vi "Init Panels.vi"(8 "error in (no error)":errorcluster, 11 "SB App in":refnum<class "SB App.lvclass">) -> (0 "error out":errorcluster, 3 "SB App out":refnum<class "SB App.lvclass">)   [LabVIEW 2020, in "SB App.lvlib" / "SB App.lvclass"]
uses:
  SB App.lvclass
  Game Config Panel/Game Config Panel.lvclass
  C:/Program Files (x86)/National Instruments/LabVIEW 2020/vi.lib/IlluminatedG/IG OOPanel/OOPanel/Panel/Panel.lvclass
  Dashboard Panel/Dashboard Panel.lvclass
  Team Field Panel/Team Field Panel.lvclass
  Square Field Panel/Square Field Panel.lvclass
  SB App.lvclass/SB App.ctl
  <vilib>/IlluminatedG/IG OOPanel/OOPanel/Manager/Manager.lvclass
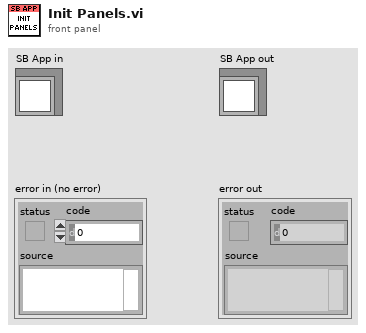
[diagram p1: front panel]
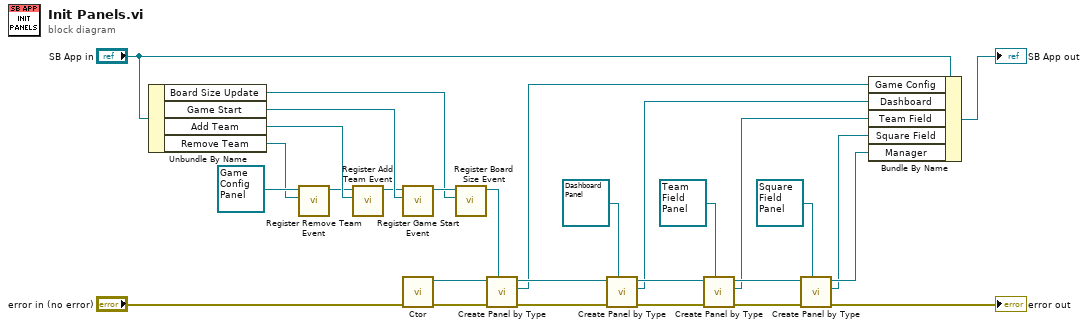
[diagram p0: block diagram]
diagram:
  n1 = Unbundle By Name("SB App in") -> ("Board Size Update"=w7:refnum<user-event>, "Game Start"=w9:refnum<user-event>, "Add Team"=w4:refnum<user-event>, "Remove Team"=w1:refnum<user-event>)
  n2 = call "Register Remove Team Event.vi"("Remove Team"=w1, "Game Config Panel in"=refnum<class "Game Config Panel.lvclass"> refnum ("SB App.lvlib:Game Config Panel.lvclass")) -> ("Game Config Panel out"=w3:refnum<class "Game Config Panel.lvclass">)  [unwired: 8 in, 1 out]
  n3 = call "Register Add Team Event.vi"("Add Team"=w4, "Game Config Panel in"=w3) -> ("Game Config Panel out"=w5:refnum<class "Game Config Panel.lvclass">)  [unwired: 8 in, 1 out]
  n4 = call "Register Game Start Event.vi"("Game Start"=w9, "Game Config Panel in"=w5) -> ("Game Config Panel out"=w8:refnum<class "Game Config Panel.lvclass">)  [unwired: 8 in, 1 out]
  n5 = call <vilib>:"Ctor.vi"("error in (no error)"="error in (no error)") -> ("error out"=w15:errorcluster, "Manager out"=w29:refnum<class "Manager.lvclass">)  [unwired: 9 in]
  n6 = call "Register Board Size Event.vi"("Board Size Update"=w7, "Game Config Panel in"=w8) -> ("Game Config Panel out"=w6:refnum<class "Game Config Panel.lvclass">)  [unwired: 8 in, 1 out]
  n7 = call <vilib>:"Create Panel by Type.vi"("Panel Type"=w6, "error in (no error)"=w15, "Manager in"=w29) -> ("error out"=w14:errorcluster, "Panel"=w18:refnum<class "Game Config Panel.lvclass">, "Manager out"=w28:refnum<class "Manager.lvclass">)  [unwired: 6 in]
  n8 = call <vilib>:"Create Panel by Type.vi"("Panel Type"=refnum<class "Dashboard Panel.lvclass"> refnum ("SB App.lvlib:Dashboard Panel.lvclass"), "error in (no error)"=w14, "Manager in"=w28) -> ("error out"=w13:errorcluster, "Panel"=w19:refnum<class "Dashboard Panel.lvclass">, "Manager out"=w25:refnum<class "Manager.lvclass">)  [unwired: 6 in]
  n9 = call <vilib>:"Create Panel by Type.vi"("Panel Type"=refnum<class "Team Field Panel.lvclass"> refnum ("SB App.lvlib:Team Field Panel.lvclass"), "error in (no error)"=w13, "Manager in"=w25) -> ("error out"=w12:errorcluster, "Panel"=w20:refnum<class "Team Field Panel.lvclass">, "Manager out"=w23:refnum<class "Manager.lvclass">)  [unwired: 6 in]
  n10 = call <vilib>:"Create Panel by Type.vi"("Panel Type"=refnum<class "Square Field Panel.lvclass"> refnum ("SB App.lvlib:Square Field Panel.lvclass"), "error in (no error)"=w12, "Manager in"=w23) -> ("error out"=→"error out":errorcluster, "Panel"=w21:refnum<class "Square Field Panel.lvclass">, "Manager out"=w22:refnum<class "Manager.lvclass">)  [unwired: 6 in]
  n11 = Bundle By Name(cluster="SB App in", "Game Config"=w18, "Dashboard"=w19, "Team Field"=w20, "Square Field"=w21, "Manager"=w22) -> (→"SB App out":refnum<class "SB App.lvclass">)
